vi "ComputeFourierPhaseOfSpecifcSF.vi"(4 "Header":T1, 6 "Col Element Number":i32, 7 "Row Element Numbert":i32, 8 "FFT size":i32=256, 9 "Scan Frame":dbl[][](array[numeric])) -> (1 "Vertical SF Phase":dbl, 3 "Horizontal SF Phase":dbl)   [LabVIEW 2012]
uses:
  <vilib>/Analysis/baseanly.llb/Mean (DBL).vi
  <vilib>/Analysis/2dsp.llb/Real FFT.vi
  <vilib>/Analysis/NI_AALPro.lvlib
  <vilib>/Analysis/NI_AALBase.lvlib
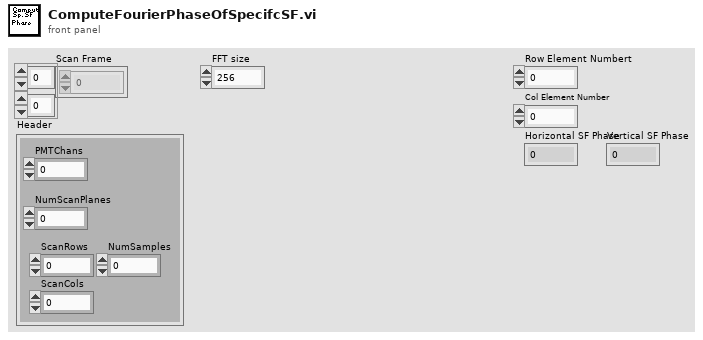
[diagram p1: front panel]
types:
  T1 = cluster{"PMTChans":i32, "NumScanPlanes":i32, "ScanRows":i32, "ScanCols":i32, "NumSamples":i32}
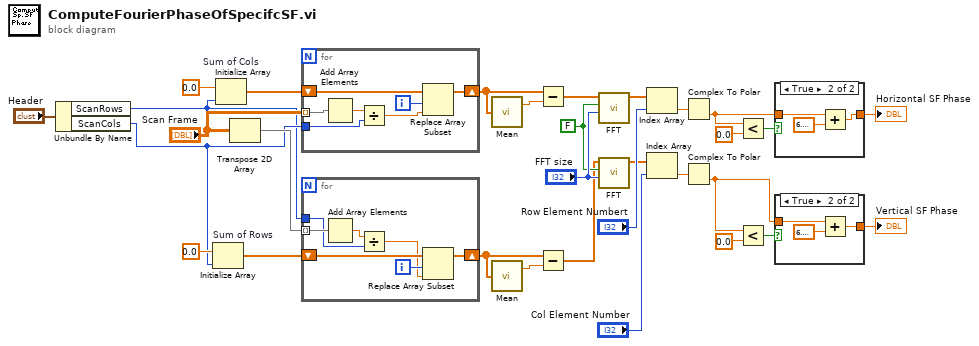
[diagram p0: block diagram]
diagram:
  w23 = FALSE ("shift?")
  n1 = Unbundle By Name("Header") -> ("ScanRows"=w1:i32, "ScanCols"=w2:i32)
  n2 = Initialize Array "Sum of Rows"(0.0 ("element"), w2) -> (w27:dbl[])
  n3 = Initialize Array "Sum of Cols"(0.0 ("element"), w1) -> (w29:dbl[])
  n4 = Transpose 2D Array(2D array="Scan Frame") -> (transposed array=w28:dbl[][])
  n5 = for {
    tunnel: "Scan Frame" -> [w38] mode=indexing
    shift-right: [w36] -> w17
    shift-left: w29 -> [w37]
    tunnel: w2 -> [w33]
    i -> [w35]
    n6 = Add Array Elements(numeric array=w38) -> (sum=w34:dbl)
    n7 = Divide(x=w34, y=w33) -> (x/y=w32:dbl)
    n8 = Replace Array Subset(array=w37, new element=w32, index=w35) -> (w36:dbl[])
  }
  n9 = for {
    tunnel: w28 -> [w45] mode=indexing
    shift-right: [w43] -> w15
    shift-left: w27 -> [w44]
    tunnel: w1 -> [w40]
    i -> [w42]
    n10 = Add Array Elements(numeric array=w45) -> (sum=w41:dbl)
    n11 = Divide(x=w41, y=w40) -> (x/y=w39:dbl)
    n12 = Replace Array Subset(array=w44, new element=w39, index=w42) -> (w43:dbl[])
  }
  n13 = call-poly <vilib>:"Mean.vi"("X"=w17) -> ("mean"=w19:dbl)  [unwired: 1 out]
  n14 = call-poly <vilib>:"Mean.vi"("X"=w15) -> ("mean"=w16:dbl)  [unwired: 1 out]
  n15 = Subtract(x=w17, y=w19) -> (x-y=w18:dbl[])
  n16 = Subtract(x=w15, y=w16) -> (x-y=w14:dbl[])
  n17 = call-poly <vilib>:"FFT.vi"("FFT size"="FFT size", "shift?"=w23, "X"=w18) -> ("FFT {X}"=w21:cdb[])  [unwired: 7 in, 1 out]
  n18 = call-poly <vilib>:"FFT.vi"("FFT size"="FFT size", "shift?"=w23, "X"=w14) -> ("FFT {X}"=w20:cdb[])  [unwired: 7 in, 1 out]
  n19 = Index Array(array=w21, index="Row Element Numbert") -> (element=w12:cdb)
  n20 = Index Array(array=w20, index="Col Element Number") -> (element=w11:cdb)
  n21 = Complex To Polar(r * e^(i*theta)=w12) -> (theta=w8:dbl)  [unwired: 1 out]
  n22 = Complex To Polar(r * e^(i*theta)=w11) -> (theta=w5:dbl)  [unwired: 1 out]
  n23 = Less?(x=w8, y=0.0) -> (x < y?=w9:bool)
  n24 = Less?(x=w5, y=0.0) -> (x < y?=w6:bool)
  n25 = case shown="True" w9 {
    tunnel: w8 -> [w46 w49]
    tunnel: [w46 w47] -> w4
    frame False {
    }
    frame True {
      n26 = Add(x=w49, y=6.283185307179586) -> (x+y=w47:dbl)
    }
  }
  "Horizontal SF Phase" <- w4
  n27 = case shown="True" w6 {
    tunnel: w5 -> [w50 w53]
    tunnel: [w50 w51] -> w3
    frame False {
    }
    frame True {
      n28 = Add(x=w53, y=6.283185307179586) -> (x+y=w51:dbl)
    }
  }
  "Vertical SF Phase" <- w3
